vi "Control Toolbar and Menubar.vi"(4 "Front Panel Window:State":T1(ring)=enum."Standard", 6 "Allow MenuBar":bool=TRUE, 8 "error in (no error)":errorcluster, 10 "Test Runtime":refnum<vi>, 11 "VI in":refnum<vi>) -> (0 "error out":errorcluster)   [LabVIEW 2017]
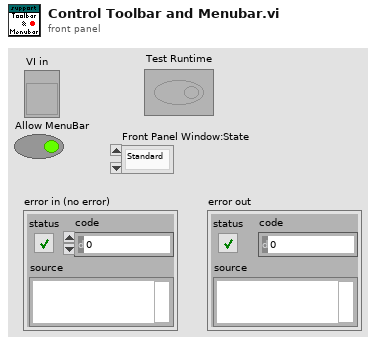
[diagram p1: front panel]
types:
  T1 = enum32{"Invalid", "Standard", "Closed", "Hidden", "Minimized", "Maximized"}
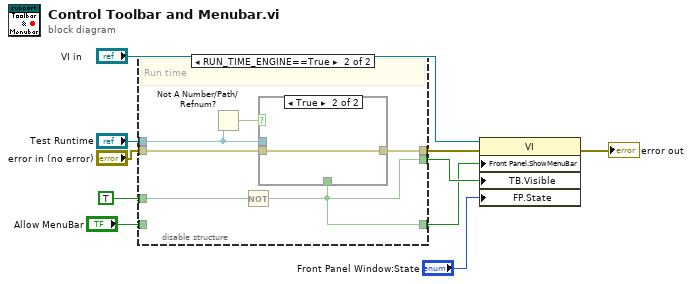
[diagram p0: block diagram]
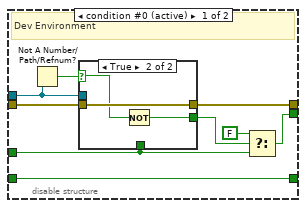
[diagram p2: hidden frame]
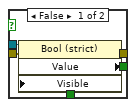
[diagram p3: hidden frame]
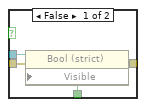
[diagram p4: hidden frame]
diagram:
  n1 = disable-structure shown="RUN_TIME_ENGINE==True" {
    disable-tunnel: [w19 w28] -> w9
    disable-tunnel: "Test Runtime" -> [w12 w30]
    disable-tunnel: TRUE -> [w16 w33]
    disable-tunnel: [w14 w32] -> w5
    disable-tunnel: "error in (no error)" -> [w15 w31]
    disable-tunnel: [w11 w28] -> w3
    disable-tunnel: "Allow MenuBar" -> [w11 _]
    frame condition #0 (active) {
      # "Dev Environment"
      n2 = Not A Number/Path/Refnum?(number/path/refnum=w12) -> (NaN/Path/Refnum?=w13:bool)
      n3 = case shown="True" w13 {
        selector: w13 -> [_ w26]
        tunnel: w12 -> [w24 _]
        tunnel: [w23 w25] -> w17
        tunnel: w16 -> [w22 _]
        tunnel: w15 -> [w21 w27]
        tunnel: [w20 w27] -> w14
        frame False {
          n4 = property class="Bool (strict)"(reference=w24, error in=w21, "Visible"=w22) -> (error out=w20:errorcluster, "Value"=w23:bool)  [unwired: 1 out]
        }
        frame True {
          n5 = Not(x=w26) -> (.not. x?=w25:bool)
        }
      }
      n6 = Select(t=FALSE, s=w17, f=w16) -> (s? t:f=w19:bool)
    }
    frame condition #1 {
      # "Run time"
      n7 = Not A Number/Path/Refnum?(number/path/refnum=w30) -> (NaN/Path/Refnum?=w29:bool)
      n8 = Not(x=w33) -> (.not. x?=w28:bool)
      n9 = case shown="True" w29 {
        tunnel: w30 -> [w37 _]
        tunnel: w28 -> [w36 _]
        tunnel: [w35 w38] -> w32
        tunnel: w31 -> [w34 w38]
        frame False {
          n10 = property class="Bool (strict)"(reference=w37, error in=w34, "Visible"=w36) -> (error out=w35:errorcluster)  [unwired: 1 out]
        }
        frame True {
        }
      }
    }
  }
  n11 = property class="VI"(reference="VI in", error in=w5, "Front Panel.ShowMenuBar"=w3, "TB.Visible"=w9, "FP.State"="Front Panel Window:State") -> (error out=→"error out":errorcluster)  [unwired: 1 out]
